vi "T281600.vi"() -> ()   [LabVIEW 2018]
uses:
  <vilib>/DAQmx/read.llb/DAQmx Read (Counter DBL 1Chan 1Samp).vi
  58b2d5aa-876a-4c16-a3d7-5584ba38aa39.vi
  c9d555a4-d372-46cd-acca-d22bdbfe3472.vi
  <vilib>/DAQmx/read.llb/DAQmx Read (Analog 1D Wfm NChan NSamp).vi
  <vilib>/DAQmx/create/channels.llb/DAQmx Create Channel (CI-Frequency).vi
  <vilib>/DAQmx/miscellaneous.llb/DAQmx Fill In Error Info.vi
  <vilib>/DAQmx/create/channels.llb/DAQmx Create Channel (AI-Voltage-Basic).vi
  <vilib>/DAQmx/configure/timing.llb/DAQmx Timing (Sample Clock).vi
  <vilib>/measure/madcrms.llb/Basic Averaged DC-RMS for N Chan.vi
  <vilib>/ptbypt/NI_PtbyPt.lvlib
  <vilib>/measure/NI_MAPro.lvlib
  <resource>/objmgr/daqmx.rc
panel:
  out "P2a":dbl format="%.1f PSI"
  out "DP3Label":string
  out "DP2Label":string
  in  "Program Select":bool
  out "ProgramName":string
  out "P2-PD (DP2) / PR-P0 (DP3)":cluster{dbl, dbl}(knob)={0.941725, 45.3733881270675} scale=0.0..550.0 scale format="%#_4f"
  out "RTD":dbl format="%.1f °F"
  out "Loop":i32
  out "Fuel Temp":dbl format="%.1f °F"
  out "FM1 Frequency":dbl format="%0.2f Hz"
  out "VSD Frequency":dbl format="%0.2f Hz"
  out "FM2 Active":bool
  out "FM1 Active":bool=TRUE
  out "?":dbl format="%.3g GPH"
  out "?":dbl(knob) scale=0.0..750.0 scale format="%#_4f"
  in  "Select FM":bool=TRUE
  out "?":dbl format="%.3g GPH"
  out "Reservoir Level":dbl(knob)=-0.5009325 scale=0.0..35.0
  out "Sol Power Volts":dbl(knob) scale=0.0..30.0
  out "TM2 Volts":dbl(knob) scale=0.0..30.0 scale format="%#.0f"
  out "TM1 Volts":dbl(knob)=-0.02039 scale=0.0..30.0
  out "Reservoir Temp":dbl(knob)=-39.01773 scale=50.0..125.0
  out "Sol Power A":dbl(knob)=-0.0872 scale=0.0..3.0
  out "TM1 mA":dbl(knob)=-0.1848 scale=0.0..2200.0 scale format="%#.1f"
  out "TM2 mA":dbl(knob)=-177.28 scale=0.0..600.0
  out "IGV (PR)":dbl(knob)=-4.7835 scale=0.0..1000.0 scale format="%#_4f"
  out "Delta P(DP1)":dbl(knob)=0.941725 scale=0.0..100.0 scale format="%#_4f"
  out "Comp Disch Pres (P8)":dbl(knob)=0.4463 scale=0.0..200.0 scale format="%#_4f"
  out "Nozzle Pres (P2/PD)":dbl(knob)=-8.992 scale=0.0..1500.0 scale format="%#_4f"
  out "Pump Disch Pres (P1)":dbl(knob)=-12.227250000000002 scale=0.0..1500.0 scale format="%#.0f"
  out "Pump Supply Pres (P0)":dbl(knob)=-1.7718 scale=0.0..200.0 scale format="%#_4f"
  in  "Stop":bool
  in  "IsFMLinear":bool
  in  "Manual Zero":bool
  in  "Tech":string
  in  "Job/PO":string
  in  "FCU PN":string="3882500"
  in  "FCU SN":string
  out "Shaft Speed":dbl(knob) scale=0.0..10000.0 scale format="%#_4f"
  out "?":dbl(knob) scale=0.0..2500.0 scale format="%#_4f"
  # "T281600 FCU Lube Pump Test System Rev 8.1"
  # "Supply Pressure"
  # "Discharge Pressure"
  # "Supply Pressure"
  # "Supply Pressure"
  # "```"
  # "Fuel Flow FM1-60"
  # "Fuel Flow FM1-20"
  # "`````"
  # "PPH x 100"
  # "PPH"
  # "Supply Pressure"
  # "Supply Pressure"
  # "```"
  # "```"
  # "```"
  # "WF"
  # "GPM"
  # "P6"
  # "DP1"
  # "Unit Data"
  # "Tech"
  # "Job #"
  # "FCU P/N"
  # "FCU S/N"
  # "Date"
  # "Time"
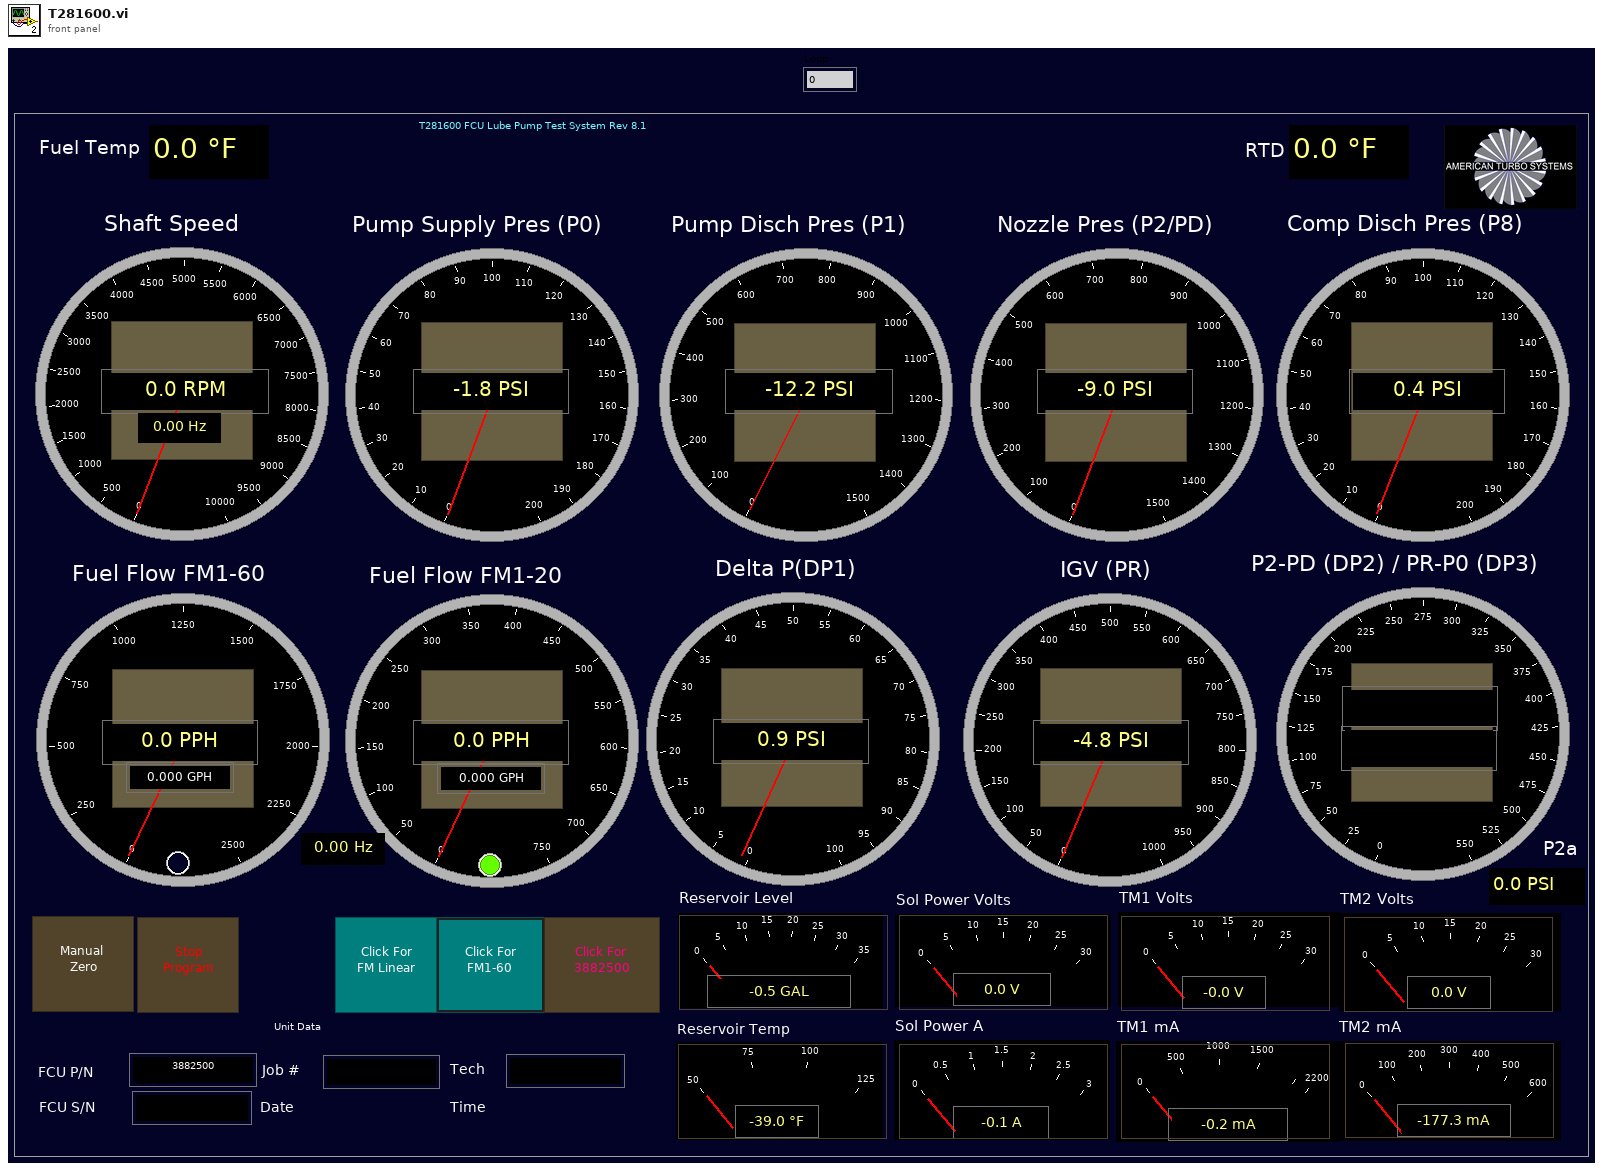
[diagram p1: front panel]
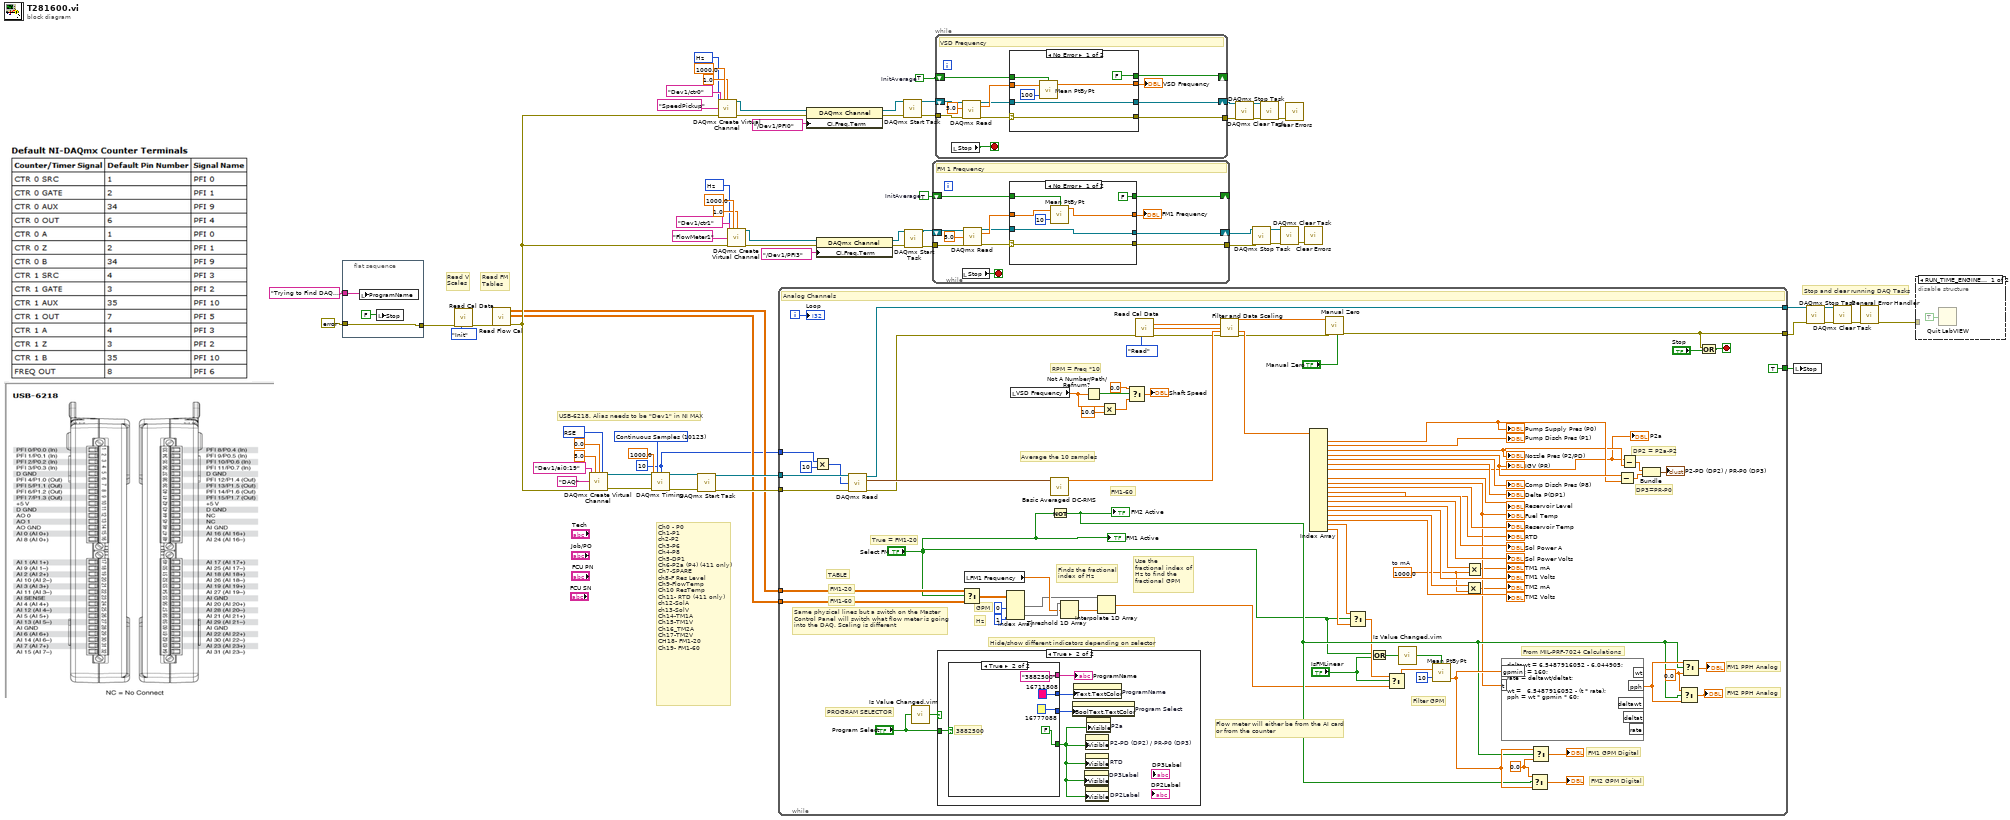
[diagram p0: block diagram]
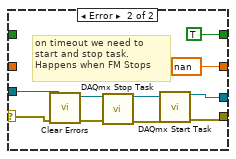
[diagram p3: hidden frame]
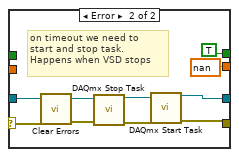
[diagram p4: hidden frame]
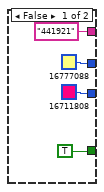
[diagram p6: hidden frame]
diagram:
  w10 = TRUE  # InitAverage
  w11 = TRUE  # InitAverage
  w20 = 10373 items=["Hz"=10373, "Ticks"=10304, "From Custom Scale"=10065] ("units")
  w21 = 10373 items=["Hz"=10373, "Ticks"=10304, "From Custom Scale"=10065] ("units")
  w3 = 10 ("samples per channel")
  w61 = 10123 items=["Finite Samples"=10178, "Continuous Samples"=10123, "Hardware Timed Single Point"=12522] ("sample mode")
  w58 = 10083 items=["Default"=-1, "RSE"=10083, "NRSE"=10078, "Differential"=10106, "Pseudodifferential"=12529] ("input terminal configuration")
  # "Ch0 - P0\nCh1-P1\nch2-P2\nCh3-P6\nCh4-P8\nCh5-DP1\nCh6-P2a (P4) (411 only)\nCh7-SPARE\nch8-F Res Level\nCh9-FlowTemp\nCh10 ResTemp\nCh11- RTD (411 only)\nch12-SolA\nch13-SolV\nCh14-TM1A\nCh15-TM1V\nCh16_TM2A\nCh17-TM2V\nCH18- FM1-20\nCh19- FM1-60"
  # "USB-6218. Alias needs to be \"Dev1\" in NI MAX"
  # "Read FM\nTables"
  # "Read V\nScales"
  # "Stop and clear running DAQ Tasks"
  n1 = flat-sequence {
    tunnel: errorcluster {"status"=FALSE, "code"=0, "source"=""} ("error in") -> [w67]
    tunnel: [w67] -> w5
    tunnel: "Trying to Find DAQ...." ("ProgramName") -> [w66]
    frame #0 {
      n2 = local write "ProgramName"(w66) -> ()
      n3 = local write "Stop"(FALSE ("stop")) -> ()
    }
  }
  n4 = call "Read Cal Data.vi"("error in (no error)"=w5, "Enum"=enum16{"Init", "Read", "Write"}."Init") -> ("error out"=w19:errorcluster)  [unwired: 1 in, 12 out]
  n5 = call "Read Flow Cal.vi"("error in"=w19) -> ("error out"=w18:errorcluster, "FM1-60"=w16:dbl[][], "FM1-20"=w17:dbl[][])  [unwired: 8 in]
  n6 = call-poly <vilib>:"DAQmx Create Virtual Channel.vi"("maximum value"=5.0, "minimum value"=0.0, "input terminal configuration"=w58, "physical channels"=tag "Dev1/ai0:19", "name to assign"="DAQ", "error in"=w18) -> ("task out"=w59:refnum<k21>, "error out"=w60:errorcluster)  [unwired: 8 in]
  n7 = call-poly <vilib>:"DAQmx Timing.vi"("task/channels in"=w59, "sample mode"=w61, "samples per channel"=w3, "rate"=1000.0, "error in"=w60) -> ("task out"=w63:refnum<k21>, "error out"=w64:errorcluster)  [unwired: 9 in]
  n8 = call <vilib>:"DAQmx Start Task.vi"("task/channels in"=w63, "error in"=w64) -> ("task out"=w54:refnum<k21>, "error out"=w50:errorcluster)  [unwired: 12 in]
  n9 = call-poly <vilib>:"DAQmx Create Virtual Channel.vi"("maximum value"=1000.0, "minimum value"=1.0, "counter"=tag "Dev1/ctr0", "name to assign"="SpeedPickup", "units"=w21, "error in"=w18) -> ("task out"=w42:refnum<k21>, "error out"=w45:errorcluster)  [unwired: 6 in, 2 out]
  n10 = call-poly <vilib>:"DAQmx Create Virtual Channel.vi"("maximum value"=1000.0, "minimum value"=1.0, "counter"=tag "Dev1/ctr1", "name to assign"="FlowMeter1", "units"=w20, "error in"=w18) -> ("task out"=w37:refnum<k21>, "error out"=w34:errorcluster)  [unwired: 6 in, 2 out]
  n11 = while {
    tunnel: w54 -> [w140]
    tunnel: [w137] -> w52
    tunnel: w17 -> [w132]
    tunnel: w16 -> [w131]
    tunnel: w50 -> [w136]
    tunnel: [w123] -> w9
    tunnel: [TRUE] -> w7
    tunnel: w3 -> [w102]
    i -> [w104]
    stop <- w122 stop-if-true
    w81 = 1000.0  # to mA
    w116 = 0.0
    w117 = 0.0
    # "Flow meter will either be from the AI card\nor from the counter"
    # "TABLE"
    # "Hide/show different indicators depending on selector"
    # "DP3=PR-P0"
    # "DP2 = P2a-P2"
    # "RPM = Freq *10"
    # "PROGRAM SELECTOR"
    # "True = FM1-20"
    # "FM1-60"
    # "Same physical lines but a switch on the Master\nControl Panel will switch what flow meter is going\ninto the DAQ. Scaling is different"
    # "FM1-60"
    # "FM1-20"
    # "Filter GPM"
    # "Use the\nfractional index of \nHz to find the \nfractional GPM"
    # "Finds the fractional\nindex of Hz"
    # "Hz"
    # "GPM"
    # "Average the 10 samples"
    # "FM2 PPH Analog"
    # "FM2 GPM Digital"
    # "From MIL-PRF-7024 Calculations"
    # "FM1 GPM Digital"
    # "FM1 PPH Analog"
    # "Analog Channels"
    n12 = Multiply(x=w102, y=10) -> (x*y=w103:i32)
    n13 = call-poly <vilib>:"DAQmx Read.vi"("task/channels in"=w140, "number of samples per channel"=w103, "error in"=w136) -> ("task out"=w137:refnum<k21>, "data"=w139:waveform(dbl)[], "error out"=w133:errorcluster)  [unwired: 10 in]
    n14 = call "Is Value Changed.vim"("value"="Program Select") -> ("changed or first call?"=w98:bool)
    n15 = case shown="True" w98 {
      tunnel: "Program Select" -> [_ w154]
      frame False {
      }
      frame True {
        n16 = case shown="True" w154 {
          tunnel: ["441921" ("ProgramName") "3882500" ("ProgramName")] -> w153
          tunnel: [u32 16777088 u32 16711808] -> w151
          tunnel: [TRUE ("Visible") FALSE ("Visible")] -> w152
          tunnel: [u32 16711808 u32 16777088] -> w150
          frame False {
          }
          frame True {
            # "3882500"
          }
        }
        "ProgramName" <- w153
        n17 = property on="Program Select" class="Bool (strict)"("BoolText.TextColor"=w150) -> ()  [unwired: 2 in, 2 out]
        n18 = property on="ProgramName" class="Str"("Text.TextColor"=w151) -> ()  [unwired: 2 in, 2 out]
        n19 = property on="DP3Label" class="Str"("Visible"=w152) -> ()  [unwired: 2 in, 2 out]
        n20 = property on="P2-PD (DP2) / PR-P0 (DP3)" class="Knob (strict)"("Visible"=w152) -> ()  [unwired: 2 in, 2 out]
        n21 = property on="RTD" class="DigNum (strict)"("Visible"=w152) -> ()  [unwired: 2 in, 2 out]
        n22 = property on="DP2Label" class="Str"("Visible"=w152) -> ()  [unwired: 2 in, 2 out]
        n23 = property on="P2a" class="DigNum (strict)"("Visible"=w152) -> ()  [unwired: 2 in, 2 out]
      }
    }
    n24 = Select(t=w132, s="Select FM", f=w131) -> (s? t:f=w130:dbl[][])
    n25 = local read "FM1 Frequency"() -> (w126:dbl)
    n26 = Index Array(array=w130, index (col) #1=0 ("disabled index (col)"), index (col) #2=1 ("index (col)")) -> (element #1=w124:dbl[], element #2=w127:dbl[])  [unwired: 2 in]
    n27 = local read "VSD Frequency"() -> (w89:dbl)
    n28 = call-poly <vilib>:"Basic Averaged DC-RMS.vi"("signals in"=w139) -> ("DC values"=w138:dbl[])  [unwired: 7 in, 3 out]
    n29 = Not(x="Select FM") -> (.not. x?=w118:bool)
    "FM2 Active" <- w118
    n30 = Threshold 1D Array(2:w126, 3:w127) -> (0:w125:dbl)  [unwired: 1 in]
    n31 = Not A Number/Path/Refnum?(number/path/refnum=w89) -> (NaN/Path/Refnum?=w87:bool)
    n32 = Interpolate 1D Array(1:w125, 2:w124) -> (0:w75:dbl)
    n33 = Multiply(x=w89, y=10.0) -> (x*y=w86:dbl)
    n34 = Select(t=0.0 ("y"), s=w87, f=w86) -> (s? t:f=→"Shaft Speed":dbl)
    n35 = call "Read Cal Data.vi"("error in (no error)"=w133, "Enum"=enum16{"Init", "Read", "Write"}."Read") -> ("Slope"=w70:dbl[], "Offset"=w134:dbl[], "error out"=w135:errorcluster)  [unwired: 1 in, 10 out]
    n36 = call "Filter and Data Scaling.vi"("Slope"=w70, "Offset"=w134, "Vin"=w138, "error in"=w135) -> ("Vout"=w79:dbl[], "ScaledOut"=w115:dbl[], "error out"=w69:errorcluster)  [unwired: 9 in]
    n37 = Index Array(array=w115) -> (element #1=w93:dbl, element #2=→"Pump Disch Pres (P1)":dbl, element #3=w92:dbl, element #4=w94:dbl, element #5=→"Comp Disch Pres (P8)":dbl, element #6=→"Delta P(DP1)":dbl, element #7=w90:dbl, element #9=→"Reservoir Level":dbl, element #10=w105:dbl, element #11=→"Reservoir Temp":dbl, element #12=→"RTD":dbl, element #13=→"Sol Power A":dbl, element #14=→"Sol Power Volts":dbl, element #15=w84:dbl, element #16=→"TM1 Volts":dbl, element #17=w82:dbl, element #18=→"TM2 Volts":dbl, element #19=w78:dbl, element #20=w77:dbl)  [unwired: 20 in, 1 out]
    "Pump Supply Pres (P0)" <- w93
    "Nozzle Pres (P2/PD)" <- w92
    "IGV (PR)" <- w94
    "Fuel Temp" <- w105
    "P2a" <- w90
    n38 = call "Manual Zero.vi"("Zero"="Manual Zero", "error in"=w69, "Vin"=w79) -> ("error out"=w123:errorcluster)  [unwired: 2 in, 6 out]
    n39 = Select(t=w78, s="Select FM", f=w77) -> (s? t:f=w76:dbl)
    n40 = Or(x="Select FM", y="IsFMLinear") -> (x .or. y?=w72:bool)
    n41 = Select(t=w76, s="IsFMLinear", f=w75) -> (s? t:f=w74:dbl)
    n42 = call "Is Value Changed.vim"("value"=w72) -> ("changed or first call?"=w120:bool)
    n43 = call <vilib>:"Mean PtByPt.vi"("x"=w74, "sample length"=10, "initialize"=w120) -> ("mean"=w143:dbl)  [unwired: 2 out]
    n44 = Multiply(x=w82, y=w81) -> (x*y=→"TM2 mA":dbl)
    n45 = Multiply(x=w84, y=w81) -> (x*y=→"TM1 mA":dbl)
    n46 = formula code="deltawt = 6.5487916052 - 6.044905;\ndeltat = 160;\nrate = deltawt/deltat;\n\nwt =   6.5487916052 - (t * rate);\npph = wt * gpmin * 60;"("gpmin"=w143, "t"=w105) -> ("pph"=w144:dbl)  [unwired: 4 out]
    n47 = Select(t=w116, s=w118, f=w143) -> (s? t:f=→"?":dbl)
    n48 = Select(t=w143, s=w118, f=w116) -> (s? t:f=→"?":dbl)
    n49 = Subtract(x=w94, y=w93) -> (x-y=w95:dbl)
    n50 = Subtract(x=w90, y=w92) -> (x-y=w91:dbl)
    n51 = Bundle(w91, w95) -> (→"P2-PD (DP2) / PR-P0 (DP3)":cluster{dbl, dbl})  [unwired: 1 in]
    n52 = Select(t=w117, s=w118, f=w144) -> (s? t:f=→"?":dbl)
    n53 = Select(t=w144, s=w118, f=w117) -> (s? t:f=→"?":dbl)
    n54 = Or(x=w123, y="Stop") -> (x .or. y?=w122:bool)
    "FM1 Active" <- "Select FM"
    "Loop" <- w104
  }
  n55 = property class="DAQmx Channel"(reference=w42, error in=w45, "CI.Freq.Term"=tag "/Dev1/PFI0" ("Frequency Input Terminal")) -> (reference out=w41:refnum<k21>, error out=w44:errorcluster)
  n56 = property class="DAQmx Channel"(reference=w37, error in=w34, "CI.Freq.Term"=tag "/Dev1/PFI3" ("Frequency Input Terminal")) -> (reference out=w38:refnum<k21>, error out=w35:errorcluster)
  n57 = call <vilib>:"DAQmx Start Task.vi"("task/channels in"=w41, "error in"=w44) -> ("task out"=w40:refnum<k21>, "error out"=w43:errorcluster)  [unwired: 12 in]
  n58 = call <vilib>:"DAQmx Start Task.vi"("task/channels in"=w38, "error in"=w35) -> ("task out"=w39:refnum<k21>, "error out"=w36:errorcluster)  [unwired: 12 in]
  n59 = while {
    tunnel: w36 -> [w173]
    tunnel: [w170] -> w13
    shift-right: [w167] -> _
    shift-left: w10 -> [w168]
    shift-right: [w165] -> w4
    shift-left: w39 -> [w174]
    stop <- w172 stop-if-true
    # "FM 1 Frequency"
    n60 = local read "Stop"() -> (w172:bool)
    n61 = call-poly <vilib>:"DAQmx Read.vi"("task/channels in"=w174, "timeout"=5.0, "error in"=w173) -> ("task out"=w166:refnum<k21>, "data"=w169:dbl, "error out"=w171:errorcluster)  [unwired: 10 in]
    n62 = case shown="No Error" w171 {
      selector: w171 -> [w181 w185]
      tunnel: [w181 w182] -> w170
      tunnel: w169 -> [w180 _]
      tunnel: [w179 nan ("data")] -> w163
      tunnel: w168 -> [w178 _]
      tunnel: [FALSE TRUE] -> w167
      tunnel: w166 -> [w175 w184]
      tunnel: [w175 w183] -> w165
      frame No Error {
        n63 = call <vilib>:"Mean PtByPt.vi"("x"=w180, "sample length"=10, "initialize"=w178) -> ("mean"=w179:dbl)  [unwired: 2 out]
      }
      frame Error {
        # "on timeout we need to \nstart and stop task.\nHappens when FM Stops"
        n64 = call <vilib>:"Clear Errors.vi"("error in (no error)"=w185) -> ("error out"=w188:errorcluster)  [unwired: 5 in, 1 out]
        n65 = call <vilib>:"DAQmx Stop Task.vi"("task/channels in"=w184, "error in"=w188) -> ("task out"=w187:refnum<k21>, "error out"=w186:errorcluster)  [unwired: 12 in]
        n66 = call <vilib>:"DAQmx Start Task.vi"("task/channels in"=w187, "error in"=w186) -> ("task out"=w183:refnum<k21>, "error out"=w182:errorcluster)  [unwired: 12 in]
      }
    }
    "FM1 Frequency" <- w163
  }
  n67 = while {
    tunnel: w43 -> [w201]
    tunnel: [w197] -> w15
    shift-right: [w194] -> _
    shift-left: w11 -> [w195]
    shift-right: [w192] -> w26
    shift-left: w40 -> [w202]
    stop <- w200 stop-if-true
    # "VSD Frequency"
    n68 = local read "Stop"() -> (w200:bool)
    n69 = call-poly <vilib>:"DAQmx Read.vi"("task/channels in"=w202, "timeout"=5.0, "error in"=w201) -> ("task out"=w193:refnum<k21>, "data"=w199:dbl, "error out"=w198:errorcluster)  [unwired: 10 in]
    n70 = case shown="No Error" w198 {
      selector: w198 -> [w209 w216]
      tunnel: w199 -> [w208 _]
      tunnel: [w209 w211] -> w197
      tunnel: [w204 nan ("data")] -> w196
      tunnel: w195 -> [w207 _]
      tunnel: [FALSE TRUE] -> w194
      tunnel: w193 -> [w205 w214]
      tunnel: [w205 w210] -> w192
      frame No Error {
        n71 = call <vilib>:"Mean PtByPt.vi"("x"=w208, "sample length"=100, "initialize"=w207) -> ("mean"=w204:dbl)  [unwired: 2 out]
      }
      frame Error {
        # "on timeout we need to \nstart and stop task.\nHappens when VSD stops"
        n72 = call <vilib>:"Clear Errors.vi"("error in (no error)"=w216) -> ("error out"=w215:errorcluster)  [unwired: 5 in, 1 out]
        n73 = call <vilib>:"DAQmx Stop Task.vi"("task/channels in"=w214, "error in"=w215) -> ("task out"=w213:refnum<k21>, "error out"=w212:errorcluster)  [unwired: 12 in]
        n74 = call <vilib>:"DAQmx Start Task.vi"("task/channels in"=w213, "error in"=w212) -> ("task out"=w210:refnum<k21>, "error out"=w211:errorcluster)  [unwired: 12 in]
      }
    }
    "VSD Frequency" <- w196
  }
  n75 = call <vilib>:"DAQmx Stop Task.vi"("task/channels in"=w26, "error in"=w15) -> ("task out"=w29:refnum<k21>, "error out"=w30:errorcluster)  [unwired: 12 in]
  n76 = call <vilib>:"DAQmx Stop Task.vi"("task/channels in"=w4, "error in"=w13) -> ("task out"=w27:refnum<k21>, "error out"=w28:errorcluster)  [unwired: 12 in]
  n77 = call <vilib>:"DAQmx Clear Task.vi"("task in"=w29, "error in"=w30) -> ("error out"=w14:errorcluster)  [unwired: 13 out]
  n78 = call <vilib>:"DAQmx Clear Task.vi"("task in"=w27, "error in"=w28) -> ("error out"=w12:errorcluster)  [unwired: 13 out]
  n79 = call <vilib>:"Clear Errors.vi"("error in (no error)"=w14) -> ()  [unwired: 5 in, 2 out]
  n80 = call <vilib>:"Clear Errors.vi"("error in (no error)"=w12) -> ()  [unwired: 5 in, 2 out]
  n81 = local write "Stop"(w7) -> ()
  n82 = call <vilib>:"DAQmx Stop Task.vi"("task/channels in"=w52, "error in"=w9) -> ("task out"=w53:refnum<k21>, "error out"=w51:errorcluster)  [unwired: 12 in]
  n83 = call <vilib>:"DAQmx Clear Task.vi"("task in"=w53, "error in"=w51) -> ("error out"=w8:errorcluster)  [unwired: 13 in]
  n84 = call <vilib>:"General Error Handler.vi"("error in (no error)"=w8) -> ("error out"=w2:errorcluster)  [unwired: 2 in, 12 out]
  n85 = disable-structure shown="RUN_TIME_ENGINE==True" {
    disable-tunnel: w2 -> [_ _]
    frame condition #0 {
      n86 = Quit LabVIEW(quit? (T)=TRUE) -> ()
    }
    frame condition #1 (active) {
    }
  }
